vi "Get visa 1d DBL data.vi"(7 "VISA resource name":refnum<visa-resource-name>, 8 "error in (no error)":errorcluster, 9 "Name":string, 10 "Mag Lab Parameters in":refnum<class "Mag Lab Parameters.lvclass">, 11 "HP87NN in":refnum<class "HP87NN.lvclass">) -> (0 "error out":errorcluster, 1 "Channel data":dbl[](array[numeric]), 2 "Channel names":string[](array[string]), 3 "HP87NN out":refnum<class "HP87NN.lvclass">, 5 "VISA resource name out":refnum<visa-resource-name>)   [LabVIEW 2015, in "HP87NN.lvclass"]
uses:
  HP87NN.lvclass
  Mag Lab Properties/Mag Lab Parameters.lvclass
  NHMFL_Core/Libraries/Instruments/GPIB/VISA  Send Receive.vi
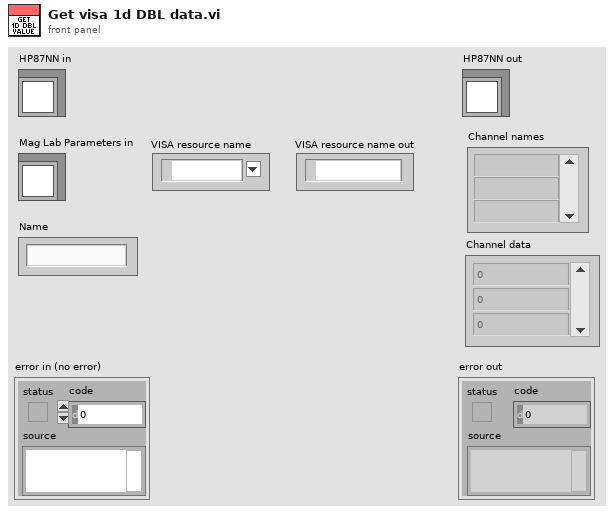
[diagram p1: front panel]
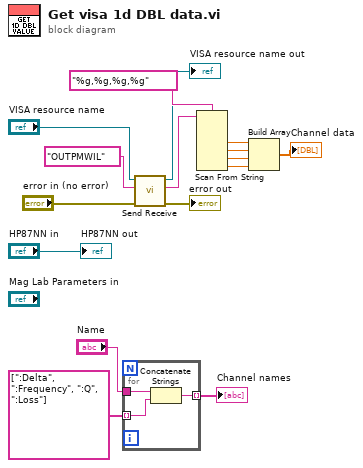
[diagram p0: block diagram]
diagram:
  n1 = for {
    tunnel: "Name" -> [w19]
    tunnel: string[] [":Delta", ":Frequency", ":Q", ":Loss"] -> [w18] mode=indexing
    tunnel: [w17] -> w14 mode=indexing
    n2 = Concatenate Strings(w19, w18) -> (w17:string)
  }
  "Channel names" <- w14
  n3 = call-poly "Send Receive.vi"("error in (no error)"="error in (no error)", "data string in"="OUTPMWIL" ("data"), "VISA Resource Name"="VISA resource name") -> ("error out"=→"error out":errorcluster, "data string out"=w10:string, "VISA Resource Name Out"=→"VISA resource name out":refnum<visa-resource-name>)  [unwired: 6 in]
  n4 = Scan From String(format string="%g,%g,%g,%g", input string=w10) -> (output 1=w8:dbl, output 2=w7:dbl, output 3=w6:dbl, output 4=w1:dbl)  [unwired: 6 in, 3 out]
  n5 = Build Array(w8, w7, w6, w1) -> (→"Channel data":dbl[])
  "HP87NN out" <- "HP87NN in"
